vi "Remove and Rewire Objects_core.vi"(8 "error in (no error)":errorcluster, 11 "Items to Remove":refnum<vi>[](array[refnum])) -> (0 "error out":errorcluster, 3 "Any Items Removed?":bool)   [LabVIEW 2017]
uses:
  <vilib>/Utility/Data Type/Type Definitions/Data Type.ctl
  <vilib>/Utility/Data Type/NI_Data Type.lvlib
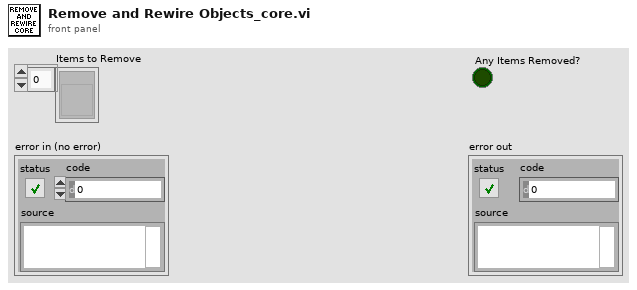
[diagram p1: front panel]
types:
  T1 = typedef "NI_Data Type.lvlib/Data Type.ctl" = enum8{"Invalid Type", "Void", "I8", "I16", "I32", "I64", "U8", "U16", "U32", "U64", "Single Float", "Double Float", "Extended Float", "Single Complex", "Double Complex", "Extended Complex", "Enum U8", "Enum U16", "Enum U32", "Enum U64", "Single Float With Unit", "Double Float With Unit", "Extended Float With Unit", "Single Complex with Unit", "Double Complex with Unit", "Extended Complex with Unit", "Boolean", "String", "Path", "Picture", "Tag", "Array", "Cluster", "Variant", "LV Variant", "Waveform", "Timestamp", "Digital Waveform", "Digital Data", "ExpressData", "Refnum", "External Data", "VI", "Poly VI", "LabVIEW Class Instance", "Fixed Point"}
  T2 = cluster{"Left":i32, "Top":i32, "Terminal":refnum<vi>}
  T3 = cluster{"Left":i32, "Top":i32, "Terminal":refnum<vi>}[]
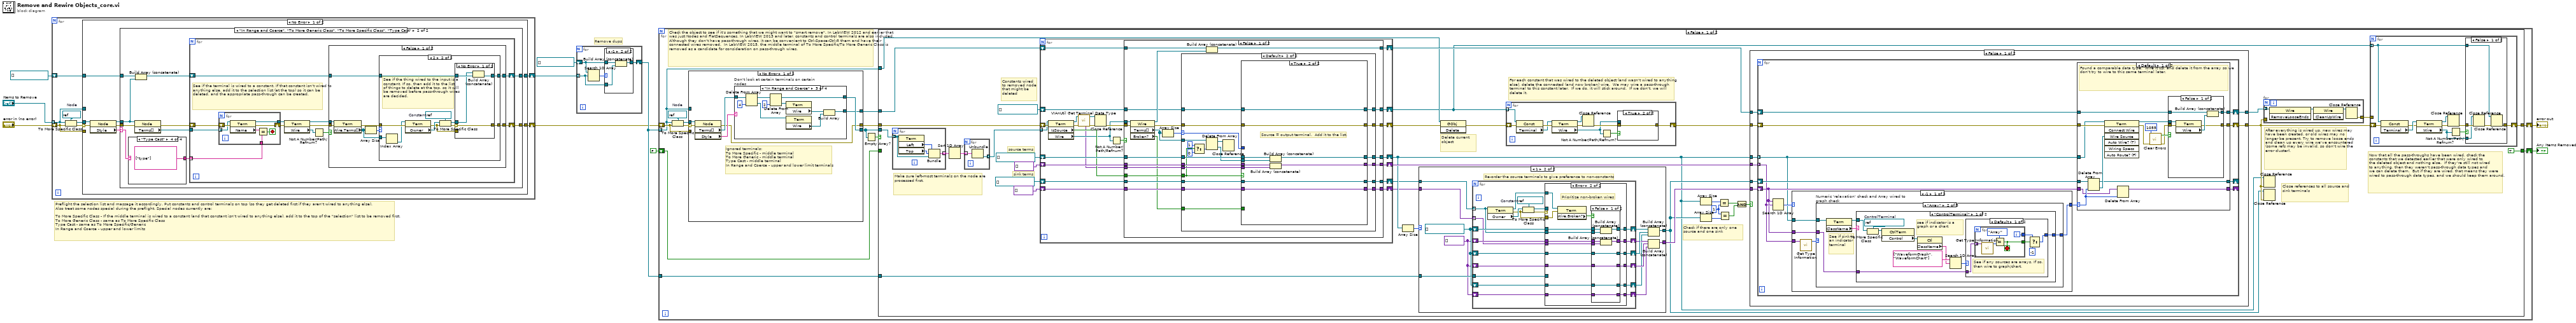
[diagram p0: block diagram]
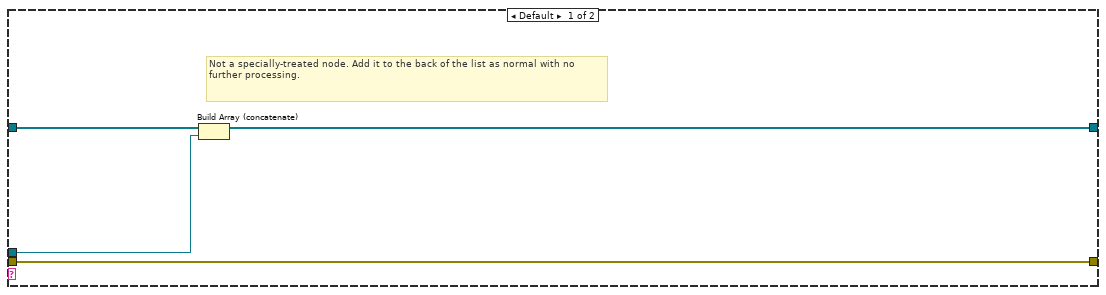
[diagram p3: hidden frame]
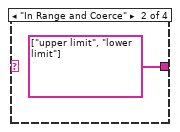
[diagram p5: hidden frame]
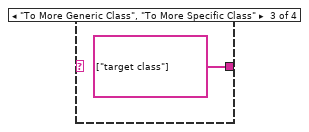
[diagram p6: hidden frame]
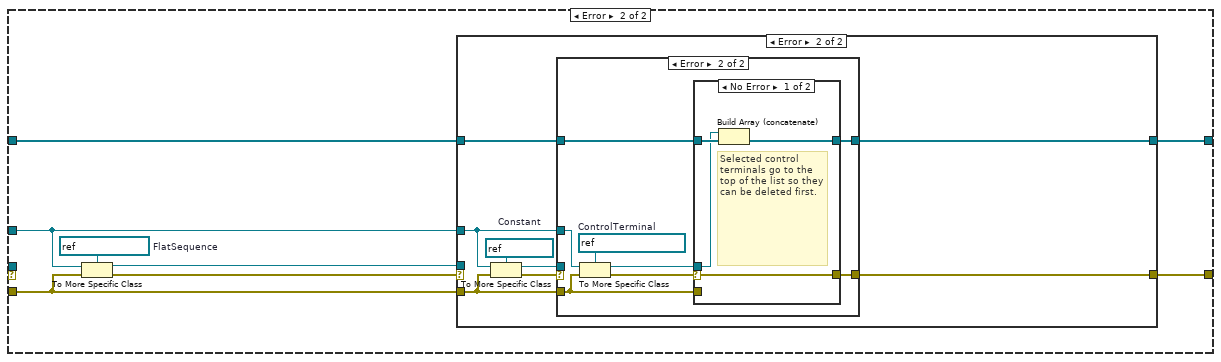
[diagram p10: hidden frame]
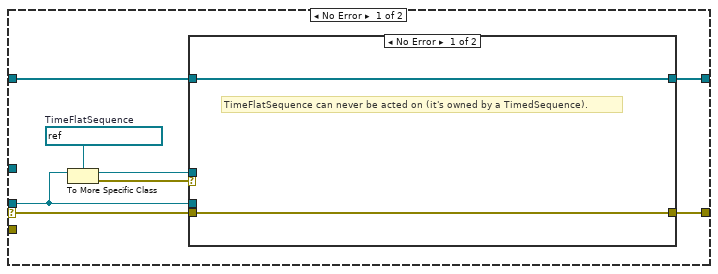
[diagram p11: hidden frame]
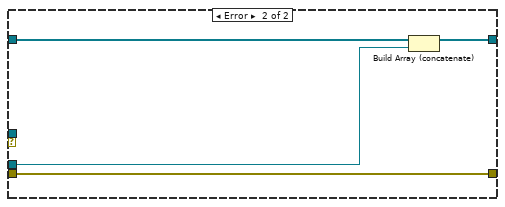
[diagram p12: hidden frame]
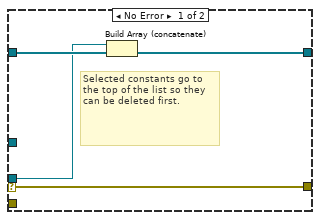
[diagram p13: hidden frame]
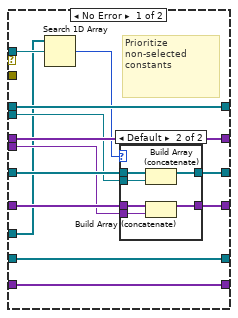
[diagram p16: hidden frame]
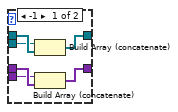
[diagram p17: hidden frame]
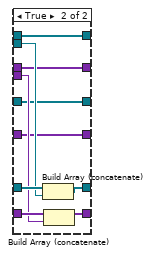
[diagram p18: hidden frame]
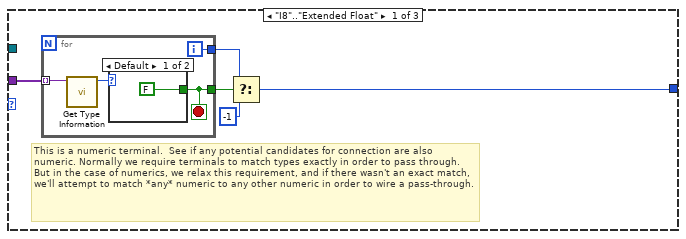
[diagram p19: hidden frame]
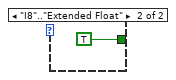
[diagram p20: hidden frame]
diagram:
  # "Preflight the selection list and massage it accordingly. Put constants and control terminals on top (so they get deleted first if they aren't wired to anything else).\nAlso treat some nodes special during the preflight. Special nodes currently are:\n\nTo More Specific Class - If the middle terminal is wired to a constant (and that constant isn't wired to anything else), add it to the top of the \"selection\" list to be removed first.\nTo More Generic Class - same as To More Specific Class\nType Cast - same as To More Specific/Generic\nIn Range and Coerce - upper and lower limits"
  # "Remove dups"
  n1 = for {
    tunnel: "Items to Remove" -> [w12] mode=indexing
    shift-right: [w13] -> w6
    shift-left: "error in (no error)" -> [w16]
    shift-right: [w14] -> w8
    shift-left: refnum<vi>[] [] ("SelList[]") -> [w15]
    w11 = refnum<vi> refnum  # Node
    n2 = To More Specific Class(target class=w11, reference=w12, error in=w16) -> (specific class reference=w18:refnum<vi>, error out=w17:errorcluster)
    n3 = case shown="No Error" w17 {
      selector: w17 -> [w26 _]
      tunnel: w18 -> [w25 _]
      tunnel: [w19 w97] -> w13
      tunnel: w12 -> [_ w95]
      tunnel: w16 -> [_ w96]
      tunnel: w15 -> [w21 w94]
      tunnel: [w20 w93] -> w14
      frame No Error {
        n4 = property class="Node"(reference=w25, error in=w26) -> (reference out=w22:refnum<vi>, error out=w23:errorcluster, "Style"=w24:string)
        n5 = case shown="\"In Range and Coerce\", \"To More Generic Class\", \"To More Specific Class\", \"Type Cast\"" w24 {
          selector: w24 -> [_ w31]
          tunnel: w23 -> [w28 w39]
          tunnel: w22 -> [w27 w38]
          tunnel: w21 -> [w30 w40]
          tunnel: [w29 w34] -> w20
          tunnel: [w28 w33] -> w19
          frame Default {
            # "Not a specially-treated node. Add it to the back of the list as normal with no further processing."
            n6 = Build Array (concatenate)(w30, w27) -> (w29:refnum<vi>[])
          }
          frame "In Range and Coerce", "To More Generic Class", "To More Specific Class", "Type Cast" {
            n7 = case shown="\"Type Cast\"" w31 {
              tunnel: [_ string[] ["upper limit", "lower limit"] string[] ["target class"] string[] ["type"]] -> w32
              frame Default {
              }
              frame "In Range and Coerce" {
              }
              frame "To More Generic Class", "To More Specific Class" {
              }
              frame "Type Cast" {
              }
            }
            n8 = property class="Node"(reference=w38, error in=w39) -> (error out=w37:errorcluster, "Terms[]"=w36:refnum<vi>[])  [unwired: 1 out]
            n9 = Build Array (concatenate)(w40, w38) -> (w35:refnum<vi>[])
            n10 = for {
              tunnel: w36 -> [w54]
              shift-right: [w50] -> w33
              shift-left: w37 -> [w55]
              shift-right: [w51] -> w34
              shift-left: w35 -> [w52]
              tunnel: w32 -> [w44] mode=indexing
              # "See if the terminal is wired to a constant. If that constant isn't wired to anything else, add it to the selection list (at the top) so it can be deleted, and the appropriate pass-through can be created."
              n11 = for {
                tunnel: w54 -> [w90] mode=indexing
                tunnel: [w88] -> w48
                shift-right: [w87] -> w53
                shift-left: w55 -> [w91]
                tunnel: w44 -> [w85]
                stop <- w86 stop-if-true
                n12 = property class="Term"(reference=w90, error in=w91) -> (reference out=w88:refnum<vi>, error out=w87:errorcluster, "Name"=w89:string)
                n13 = Equal?(x=w89, y=w85) -> (x = y?=w86:bool)
              }
              n14 = property class="Term"(reference=w48, error in=w53) -> (reference out=w47:refnum<vi>, error out=w49:errorcluster, "Wire"=w46:refnum<vi>)
              n15 = Not A Number/Path/Refnum?(number/path/refnum=w46) -> (NaN/Path/Refnum?=w45:bool)
              n16 = case shown="False" w45 {
                tunnel: w52 -> [w63 w84]
                tunnel: [w60 w84] -> w51
                tunnel: [w59 w83] -> w50
                tunnel: w49 -> [w57 w83]
                tunnel: w47 -> [w56 _]
                frame False {
                  n17 = property class="Term"(reference=w56, error in=w57) -> (error out=w62:errorcluster, "Wire.Terms[]"=w58:refnum<vi>[])  [unwired: 1 out]
                  n18 = Array Size(array=w58) -> (size(s)=w61:i32)
                  n19 = case shown="2" w61 {
                    tunnel: w63 -> [w65 w70]
                    tunnel: w62 -> [w64 w75]
                    tunnel: [w65 w69] -> w60
                    tunnel: [w64 w67] -> w59
                    tunnel: w58 -> [_ w76]
                    frame Default {
                      # "Any number of terminals on the upper/lower limit wires other than 2 means that whatever is wired to it, is also wired to something else. Don't try to delete that thing in this case."
                    }
                    frame 2 {
                      w72 = refnum<vi> refnum  # Constant
                      # "See if the thing wired to the input is a constant. If so, then add it to the list of things to delete at the top, so it will be removed before pass-through wires are decided."
                      n20 = Index Array(array=w76) -> (element=w74:refnum<vi>)  [unwired: 1 in]
                      n21 = property class="Term"(reference=w74, error in=w75) -> (error out=w68:errorcluster, "Owner"=w73:refnum<vi>)  [unwired: 1 out]
                      n22 = To More Specific Class(target class=w72, reference=w73, error in=w68) -> (specific class reference=w66:refnum<vi>, error out=w71:errorcluster)
                      n23 = case shown="No Error" w71 {
                        selector: w71 -> [w78 _]
                        tunnel: w70 -> [w80 w82]
                        tunnel: [w79 w82] -> w69
                        tunnel: w68 -> [_ w81]
                        tunnel: [w78 w81] -> w67
                        tunnel: w66 -> [w77 _]
                        frame No Error {
                          n24 = Build Array (concatenate)(w77, w80) -> (w79:refnum<vi>[])
                        }
                        frame Error {
                        }
                      }
                    }
                  }
                }
                frame True {
                  # "Terminal is not wired...no further work necessary"
                }
              }
            }
          }
        }
      }
      frame Error {
        w92 = refnum<vi> refnum  # FlatSequence
        n25 = To More Specific Class(target class=w92, reference=w95, error in=w96) -> (specific class reference=w98:refnum<vi>, error out=w99:errorcluster)
        n26 = case shown="Error" w99 {
          selector: w99 -> [w102 _]
          tunnel: w98 -> [w104 _]
          tunnel: [w101 w117] -> w97
          tunnel: w96 -> [_ w118]
          tunnel: w95 -> [_ w119]
          tunnel: w94 -> [w107 w116]
          tunnel: [w106 w115] -> w93
          frame No Error {
            w105 = refnum<vi> refnum  # TimeFlatSequence
            n27 = To More Specific Class(target class=w105, reference=w104) -> (specific class reference=w100:refnum<vi>, error out=w103:errorcluster)  [unwired: 1 in]
            n28 = case shown="No Error" w103 {
              tunnel: w107 -> [w108 w113]
              tunnel: [w108 w112] -> w106
              tunnel: w104 -> [_ w111]
              tunnel: w102 -> [w109 w110]
              tunnel: [w109 w110] -> w101
              tunnel: w100 -> [_ _]
              frame No Error {
                # "TimeFlatSequence can never be acted on (it's owned by a TimedSequence)."
              }
              frame Error {
                n29 = Build Array (concatenate)(w113, w111) -> (w112:refnum<vi>[])
              }
            }
          }
          frame Error {
            w114 = refnum<vi> refnum  # Constant
            n30 = To More Specific Class(target class=w114, reference=w119, error in=w118) -> (specific class reference=w120:refnum<vi>, error out=w121:errorcluster)
            n31 = case shown="Error" w121 {
              selector: w121 -> [w125 _]
              tunnel: w120 -> [w122 _]
              tunnel: w119 -> [_ w133]
              tunnel: w118 -> [_ w130]
              tunnel: [w125 w129] -> w117
              tunnel: w116 -> [w124 w128]
              tunnel: [w123 w127] -> w115
              frame No Error {
                # "Selected constants go to the top of the list so they can be deleted first."
                n32 = Build Array (concatenate)(w122, w124) -> (w123:refnum<vi>[])
              }
              frame Error {
                w126 = refnum<vi> refnum  # ControlTerminal
                n33 = To More Specific Class(target class=w126, reference=w133, error in=w130) -> (specific class reference=w131:refnum<vi>, error out=w132:errorcluster)
                n34 = case shown="No Error" w132 {
                  selector: w132 -> [w137 _]
                  tunnel: w131 -> [w134 _]
                  tunnel: w130 -> [_ w139]
                  tunnel: [w137 w139] -> w129
                  tunnel: w128 -> [w136 w138]
                  tunnel: [w135 w138] -> w127
                  frame No Error {
                    # "Selected control terminals go to the top of the list so they can be deleted first."
                    n35 = Build Array (concatenate)(w134, w136) -> (w135:refnum<vi>[])
                  }
                  frame Error {
                  }
                }
              }
            }
          }
        }
      }
    }
  }
  n36 = for {
    tunnel: w8 -> [w140] mode=indexing
    shift-right: [w141] -> w10
    shift-left: refnum<vi>[] [] ("SelList[]") -> [w142]
    n37 = Search 1D Array(1D array=w142, element=w140) -> (index of element=w143:i32)  [unwired: 1 in]
    n38 = case shown="-1" w143 {
      tunnel: w142 -> [w144 w147]
      tunnel: [w144 w146] -> w141
      tunnel: w140 -> [_ w145]
      frame Default {
      }
      frame -1 {
        n39 = Build Array (concatenate)(w147, w145) -> (w146:refnum<vi>[])
      }
    }
  }
  n40 = for {
    tunnel: w10 -> [w154] mode=indexing
    shift-right: [w153] -> w2
    shift-left: FALSE -> [w148]
    shift-right: [w152] -> w3
    shift-left: w6 -> [w158]
    tunnel: w10 -> [w151]
    w150 = refnum<vi> refnum  # Node
    # "Check the object to see if it's something that we might want to \"smart remove\". In LabVIEW 2012 and earlier that was just Nodes and FlatSequences. In LabVIEW 2013 and later, constants and control terminals are also included. Although they don't have pass-through wires, it can be convenient to Ctrl-Space-Ctrl-R them and have their connected wires removed.  In LabVIEW 2015, the middle terminal of To More Specific/To More Generic Class is removed as a candidate for consideration on pass-through wires."
    n41 = To More Specific Class(target class=w150, reference=w154, error in=w158) -> (specific class reference=w159:refnum<vi>, error out=w160:errorcluster)
    n42 = case shown="No Error" w160 {
      selector: w160 -> [w572 _]
      tunnel: w159 -> [w571 _]
      tunnel: [w568 w598] -> w155
      tunnel: [w566 w600] -> w156
      tunnel: w154 -> [_ w597]
      tunnel: w158 -> [_ w599]
      tunnel: [w567 _] -> w149
      frame No Error {
        # "Ignored terminals:\nTo More Specific - middle terminal\nTo More Generic - middle terminal\nType Cast - middle terminal\nIn Range and Coerce - upper and lower limit terminals"
        n43 = property class="Node"(reference=w571, error in=w572) -> (error out=w566:errorcluster, "Terms[]"=w569:refnum<vi>[], "Style"=w570:string)  [unwired: 1 out]
        n44 = case "Don't look at certain terminals on certain nodes" shown="\"In Range and Coerce\"" w570 {
          tunnel: w569 -> [w578 w584 w594 w595]
          tunnel: [w576 w582 w588 w595] -> w568
          tunnel: [w573 w579 w590 _] -> w567
          frame "To More Generic Class", "Type Cast" {
            n45 = Delete From Array(array=w578, index=1) -> (deleted portion=w574:refnum<vi>, array with subset deleted=w576:refnum<vi>[])  [unwired: 1 in]
            n46 = property class="Term"(reference=w574) -> ("Wire"=w575:refnum<vi>)  [unwired: 1 in, 2 out]
            n47 = Build Array(w575) -> (w573:refnum<vi>[])
          }
          frame "To More Specific Class" {
            n48 = Delete From Array(array=w584, index=2) -> (deleted portion=w580:refnum<vi>, array with subset deleted=w582:refnum<vi>[])  [unwired: 1 in]
            n49 = property class="Term"(reference=w580) -> ("Wire"=w581:refnum<vi>)  [unwired: 1 in, 2 out]
            n50 = Build Array(w581) -> (w579:refnum<vi>[])
          }
          frame "In Range and Coerce" {
            n51 = Delete From Array(array=w594, index=4) -> (deleted portion=w591:refnum<vi>, array with subset deleted=w589:refnum<vi>[])  [unwired: 1 in]
            n52 = Delete From Array(array=w589, index=2) -> (deleted portion=w586:refnum<vi>, array with subset deleted=w588:refnum<vi>[])  [unwired: 1 in]
            n53 = property class="Term"(reference=w586) -> ("Wire"=w585:refnum<vi>)  [unwired: 1 in, 2 out]
            n54 = property class="Term"(reference=w591) -> ("Wire"=w592:refnum<vi>)  [unwired: 1 in, 2 out]
            n55 = Build Array(w585, w592) -> (w590:refnum<vi>[])
          }
          frame Default {
          }
        }
      }
      frame Error {
        w596 = refnum<vi> refnum  # FlatSequence
        n56 = To More Specific Class(target class=w596, reference=w597, error in=w599) -> (specific class reference=w601:refnum<vi>, error out=w602:errorcluster)
        n57 = case shown="Error" w602 {
          selector: w602 -> [w606 _]
          tunnel: w601 -> [w605 _]
          tunnel: [w604 w608] -> w600
          tunnel: w599 -> [_ w610]
          tunnel: [w603 w609] -> w598
          tunnel: w597 -> [_ w611]
          frame No Error {
            n58 = property class="FlatSeq"(reference=w605, error in=w606) -> (error out=w604:errorcluster, "Terms[]"=w603:refnum<vi>[])  [unwired: 1 out]
          }
          frame Error {
            w607 = refnum<vi> refnum  # Constant
            n59 = To More Specific Class(target class=w607, reference=w611, error in=w610) -> (specific class reference=w612:refnum<vi>, error out=w613:errorcluster)
            n60 = case shown="Error" w613 {
              selector: w613 -> [w617 _]
              tunnel: w612 -> [w618 _]
              tunnel: w611 -> [_ w625]
              tunnel: w610 -> [_ w622]
              tunnel: [w615 w620] -> w609
              tunnel: [w614 w621] -> w608
              frame No Error {
                n61 = property class="Const"(reference=w618, error in=w617) -> (error out=w614:errorcluster, "Terminal"=w616:refnum<vi>)  [unwired: 1 out]
                n62 = Build Array(w616) -> (w615:refnum<vi>[])
              }
              frame Error {
                w619 = refnum<vi> refnum  # ControlTerminal
                n63 = To More Specific Class(target class=w619, reference=w625, error in=w622) -> (specific class reference=w623:refnum<vi>, error out=w624:errorcluster)
                n64 = case shown="No Error" w624 {
                  selector: w624 -> [w628 _]
                  tunnel: w623 -> [w627 _]
                  tunnel: w622 -> [_ w629]
                  tunnel: [w628 w629] -> w621
                  tunnel: [w626 _] -> w620
                  frame No Error {
                    n65 = Build Array(w627) -> (w626:refnum<vi>[])
                  }
                  frame Error {
                  }
                }
              }
            }
          }
        }
      }
    }
    n66 = Empty Array?(array=w155) -> (empty?=w157:bool)
    n67 = case shown="False" w157 {
      tunnel: w156 -> [w196 w565]
      tunnel: [w182 w565] -> w152
      tunnel: w148 -> [_ w564]
      tunnel: w155 -> [w163 _]
      tunnel: w154 -> [w186 _]
      tunnel: [TRUE w564] -> w153
      tunnel: w151 -> [w168 _]
      tunnel: w149 -> [w161 _]
      frame False {
        w177 = 1 ("y")
        # "Make sure left-most terminals on the node are processed first."
        # "Check if there are only one source and one sink"
        # "Now that all the pass-throughs have been wired, check the\nconstants that we detected earlier that were only wired to\nthe deleted object and nothing else.  If they're still not wired\nto anything, then they weren't pass-through data types and\nwe can delete them.  But if they are wired, that means they were\nwired to pass-through data types, and we should keep them around."
        # "For each constant that was wired to the deleted object (and wasn't wired to anything\nelse), delete the connected (and now broken) wire.  We may wire a pass-through\nterminal to this constant later.  If we do, it will stick around.  If we don't, we will\ndelete it."
        # "Constants wired\nto removed node\nthat might be\ndeleted"
        # "After everything is wired up, new wires may have been created, or old wires may no longer be present. Try to remove loose ends and clean up every wire we've encountered (some refs may be invalid, so don't wire the error cluster)."
        # "Close references to all source and\nsink terminals"
        # "Delete current object"
        # "sink terms"
        # "source terms"
        n68 = for {
          tunnel: w163 -> [w200] mode=indexing
          tunnel: [w201] -> w165 mode=indexing
          n69 = property class="Term"(reference=w200) -> ("Left"=w202:i32, "Top"=w199:i32)  [unwired: 1 in, 2 out]
          n70 = Bundle("Left"=w202, "Top"=w199, "Terminal"=w200) -> (w201:T2)  [unwired: 1 in]
        }
        n71 = Sort 1D Array(array=w165) -> (sorted array=w164:T3)
        n72 = for {
          tunnel: w164 -> [w198] mode=indexing
          tunnel: [w197] -> w162 mode=indexing
          n73 = Unbundle(w198) -> ("Terminal"=w197:refnum<vi>)  [unwired: 2 out]
        }
        n74 = for {
          shift-right: [w451] -> w190
          shift-left: w196 -> [w463]
          tunnel: w162 -> [w462] mode=indexing
          shift-right: [w455] -> w170
          shift-left: refnum<vi>[] [] -> [w461]
          shift-right: [w454] -> w173
          shift-left: variant[] [] -> [w460]
          shift-right: [w457] -> w167
          shift-left: refnum<vi>[] [] -> [w459]
          shift-right: [w456] -> w166
          shift-left: variant[] [] -> [w458]
          shift-right: [w447] -> w189
          shift-left: w161 -> [w448]
          shift-right: [w445] -> w180
          shift-left: refnum<vi>[] [] -> [w446]
          n75 = property class="Term"(reference=w462, error in=w463) -> (reference out=w442:refnum<vi>, error out=w444:errorcluster, "IsSource"=w452:bool, "Wire"=w450:refnum<vi>)
          n76 = call <vilib>:"VIAnUtil Get Terminal Data Type.vi"("error in (no error)"=w444, "Terminal"=w442) -> ("error out"=w443:errorcluster, "dup  Terminal"=w441:refnum<vi>, "Type Variant"=w440:variant)  [unwired: 6 in, 1 out]
          n77 = Close Reference(reference=w441, error in (no error)=w443) -> (error out=w453:errorcluster)
          n78 = Not A Number/Path/Refnum?(number/path/refnum=w450) -> (NaN/Path/Refnum?=w449:bool)
          n79 = case shown="False" w449 {
            tunnel: w461 -> [w485 w561]
            tunnel: w460 -> [w484 w560]
            tunnel: w459 -> [w483 w559]
            tunnel: w458 -> [w482 w558]
            tunnel: w440 -> [w481 _]
            tunnel: [w480 w559] -> w457
            tunnel: [w479 w558] -> w456
            tunnel: [w478 w561] -> w455
            tunnel: [w477 w560] -> w454
            tunnel: w453 -> [w476 w562]
            tunnel: w452 -> [w474 _]
            tunnel: [w468 w562] -> w451
            tunnel: w450 -> [w475 _]
            tunnel: w448 -> [w473 w563]
            tunnel: [w472 w563] -> w447
            tunnel: w446 -> [w469 w557]
            tunnel: [w467 w557] -> w445
            frame False {
              n80 = property class="Wire"(reference=w475, error in=w476) -> (reference out=w471:refnum<vi>, error out=w470:errorcluster, "Terms[]"=w466:refnum<vi>[], "Broken?"=w464:bool)
              n81 = Array Size(array=w466) -> (size(s)=w465:i32)
              n82 = case shown="Default" w465 {
                selector: w465 -> [_ w494]
                tunnel: w485 -> [w489 w514]
                tunnel: w484 -> [w490 w513]
                tunnel: w483 -> [w491 w512]
                tunnel: w482 -> [w492 w511]
                tunnel: w481 -> [_ w510]
                tunnel: [w491 w509] -> w480
                tunnel: [w492 w508] -> w479
                tunnel: [w489 w507] -> w478
                tunnel: [w490 w506] -> w477
                tunnel: w474 -> [_ w500]
                tunnel: w470 -> [w486 w499]
                tunnel: w469 -> [w488 w498]
                tunnel: [w486 w497] -> w468
                tunnel: [w488 w496] -> w467
                tunnel: w466 -> [w487 w495]
                tunnel: w464 -> [_ w493]
                frame 1 {
                  # "If the wire only has one terminal, then it is a broken wire, with either no source\nor no sink.  Don't try to get data type information on this wire, as it will end up\nbeing removed by the \"Remove Loose Ends\" call later (note that we're still adding\nthe wire to the wires array above)."
                  n83 = Close Reference(reference=w487) -> ()  [unwired: 1 in, 1 out]
                }
                frame Default {
                  n84 = Select(t=1, s=w500, f=0) -> (s? t:f=w503:i32)
                  n85 = Delete From Array(array=w495, index=w503) -> (deleted portion=w501:refnum<vi>, array with subset deleted=w502:refnum<vi>[])  [unwired: 1 in]
                  n86 = Close Reference(reference=w502) -> ()  [unwired: 1 in, 1 out]
                  n87 = case shown="True" w500 {
                    tunnel: w514 -> [w533 w554]
                    tunnel: w513 -> [w532 w552]
                    tunnel: w512 -> [w535 w556]
                    tunnel: w511 -> [w534 w555]
                    tunnel: w510 -> [w518 w549]
                    tunnel: w501 -> [w521 w553]
                    tunnel: [w531 w556] -> w509
                    tunnel: [w530 w555] -> w508
                    tunnel: [w533 w551] -> w507
                    tunnel: [w532 w550] -> w506
                    tunnel: w499 -> [w529 w548]
                    tunnel: w498 -> [w523 w547]
                    tunnel: [w524 w548] -> w497
                    tunnel: [w522 w547] -> w496
                    tunnel: w494 -> [w520 _]
                    tunnel: w493 -> [w519 _]
                    frame False {
                      w515 = refnum<vi> refnum  # Constant
                      # "If wire was broken, use data type of source term (instead of sink on removed item) when trying to make a match later."
                      # "Sink = input terminal.  Add it to the list, and if it's wired to a constant, add that to the list of constants to potentially delete.  Except if the constant is wired to something else... in that case, keep the const."
                      n88 = property class="Term"(reference=w521, error in=w529) -> (error out=w525:errorcluster, "Owner"=w528:refnum<vi>, "Data Type"=w516:variant)  [unwired: 1 out]
                      n89 = Select(t=w516, s=w519, f=w518) -> (s? t:f=w517:variant)
                      n90 = To More Specific Class(target class=w515, reference=w528, error in=w525) -> (specific class reference=w526:refnum<vi>, error out=w527:errorcluster)
                      n91 = case shown="No Error" w527 {
                        selector: w527 -> [w538 _]
                        tunnel: w526 -> [w537 _]
                        tunnel: w525 -> [_ w546]
                        tunnel: [w538 w546] -> w524
                        tunnel: [w539 w545] -> w522
                        tunnel: w523 -> [w540 w545]
                        tunnel: w520 -> [w536 _]
                        frame No Error {
                          n92 = case shown="..2" w536 {
                            tunnel: w540 -> [w541 w544]
                            tunnel: [w541 w543] -> w539
                            tunnel: w537 -> [_ w542]
                            frame 3.. {
                            }
                            frame ..2 {
                              n93 = Build Array (concatenate)(w544, w542) -> (w543:refnum<vi>[])
                            }
                          }
                        }
                        frame Error {
                        }
                      }
                      n94 = Build Array (concatenate)(w535, w521) -> (w531:refnum<vi>[])
                      n95 = Build Array (concatenate)(w534, w517) -> (w530:variant[])
                    }
                    frame True {
                      # "Source = output terminal.  Add it to the list."
                      n96 = Build Array (concatenate)(w554, w553) -> (w551:refnum<vi>[])
                      n97 = Build Array (concatenate)(w552, w549) -> (w550:variant[])
                    }
                  }
                }
              }
              n98 = Build Array (concatenate)(w473, w471) -> (w472:refnum<vi>[])
            }
            frame True {
              # "This terminal isn't wired to anything.  Ignore it."
            }
          }
        }
        n99 = Array Size(array=w170) -> (size(s)=w169:i32)
        n100 = case shown="1" w169 {
          tunnel: w167 -> [w204 w217]
          tunnel: w166 -> [w203 w216]
          tunnel: [w203 w215] -> w172
          tunnel: [w204 w214] -> w171
          tunnel: w168 -> [_ w209]
          frame Default {
          }
          frame 1 {
            w207 = variant[] []
            w208 = refnum<vi>[] []
            # "Re-order the source terminals to give preference to non-constants"
            n101 = for {
              tunnel: w217 -> [w229] mode=indexing
              tunnel: w216 -> [w230] mode=indexing
              shift-right: [w232] -> w213
              shift-left: w208 -> [w234]
              shift-right: [w231] -> w211
              shift-left: w207 -> [w233]
              shift-right: [w227] -> w212
              shift-left: w208 -> [w228]
              shift-right: [w225] -> w210
              shift-left: w207 -> [w226]
              tunnel: w209 -> [w224]
              shift-right: [w219] -> w206
              shift-left: w208 -> [w221]
              shift-right: [w218] -> w205
              shift-left: w207 -> [w220]
              w237 = refnum<vi> refnum  # Constant
              n102 = property class="Term"(reference=w229) -> (reference out=w223:refnum<vi>, error out=w222:errorcluster, "Owner"=w238:refnum<vi>)  [unwired: 1 in]
              n103 = To More Specific Class(target class=w237, reference=w238, error in=w222) -> (specific class reference=w235:refnum<vi>, error out=w236:errorcluster)
              n104 = case shown="Error" w236 {
                tunnel: w235 -> [w243 _]
                tunnel: w234 -> [w251 w280]
                tunnel: w233 -> [w250 w279]
                tunnel: [w251 w278] -> w232
                tunnel: [w250 w277] -> w231
                tunnel: w230 -> [w244 w276]
                tunnel: w229 -> [w248 w275]
                tunnel: [w247 w266] -> w227
                tunnel: w228 -> [w249 w267]
                tunnel: w226 -> [w246 w265]
                tunnel: [w245 w264] -> w225
                tunnel: w224 -> [w242 _]
                tunnel: w223 -> [_ w273]
                tunnel: w222 -> [_ w274]
                tunnel: w221 -> [w240 w270]
                tunnel: w220 -> [w239 w268]
                tunnel: [w240 w271] -> w219
                tunnel: [w239 w269] -> w218
                frame No Error {
                  # "Prioritize non-selected constants"
                  n105 = Search 1D Array(1D array=w242, element=w243) -> (index of element=w241:i32)  [unwired: 1 in]
                  n106 = case shown="Default" w241 {
                    tunnel: w249 -> [w257 w263]
                    tunnel: w248 -> [w256 w262]
                    tunnel: [w255 w261] -> w247
                    tunnel: w246 -> [w254 w260]
                    tunnel: [w253 w259] -> w245
                    tunnel: w244 -> [w252 w258]
                    frame -1 {
                      n107 = Build Array (concatenate)(w256, w257) -> (w255:refnum<vi>[])
                      n108 = Build Array (concatenate)(w252, w254) -> (w253:variant[])
                    }
                    frame Default {
                      n109 = Build Array (concatenate)(w263, w262) -> (w261:refnum<vi>[])
                      n110 = Build Array (concatenate)(w260, w258) -> (w259:variant[])
                    }
                  }
                }
                frame Error {
                  # "Prioritize non-broken wires"
                  n111 = property class="Term"(reference=w273, error in=w274) -> ("Wire.Broken?"=w272:bool)  [unwired: 2 out]
                  n112 = case shown="False" w272 {
                    tunnel: w280 -> [w290 w294]
                    tunnel: w279 -> [w287 w293]
                    tunnel: [w289 w294] -> w278
                    tunnel: [w286 w293] -> w277
                    tunnel: w276 -> [w285 w295]
                    tunnel: w275 -> [w288 w298]
                    tunnel: [w284 w300] -> w271
                    tunnel: w270 -> [w284 w299]
                    tunnel: [w283 w297] -> w269
                    tunnel: w268 -> [w283 w296]
                    tunnel: w267 -> [w282 w292]
                    tunnel: [w282 w292] -> w266
                    tunnel: w265 -> [w281 w291]
                    tunnel: [w281 w291] -> w264
                    frame False {
                      n113 = Build Array (concatenate)(w290, w288) -> (w289:refnum<vi>[])
                      n114 = Build Array (concatenate)(w287, w285) -> (w286:variant[])
                    }
                    frame True {
                      n115 = Build Array (concatenate)(w299, w298) -> (w300:refnum<vi>[])
                      n116 = Build Array (concatenate)(w296, w295) -> (w297:variant[])
                    }
                  }
                }
              }
            }
            n117 = Build Array (concatenate)(w213, w212, w206) -> (w214:refnum<vi>[])
            n118 = Build Array (concatenate)(w211, w210, w205) -> (w215:variant[])
          }
        }
        n119 = invoke class="GObj" method="Delete"(reference=w186, error in=w190) -> (error out=w185:errorcluster)  [unwired: 1 in, 2 out]
        n120 = for {
          tunnel: w180 -> [w430] mode=indexing
          shift-right: [w424] -> w184
          shift-left: w185 -> [w431]
          n121 = property class="Const"(reference=w430, error in=w431) -> (error out=w429:errorcluster, "Terminal"=w428:refnum<vi>)  [unwired: 1 out]
          n122 = property class="Term"(reference=w428, error in=w429) -> (reference out=w426:refnum<vi>, error out=w427:errorcluster, "Wire"=w423:refnum<vi>)
          n123 = Close Reference(reference=w426, error in (no error)=w427) -> (error out=w425:errorcluster)
          n124 = Not A Number/Path/Refnum?(number/path/refnum=w423) -> (NaN/Path/Refnum?=w422:bool)
          n125 = case shown="True" w422 {
            tunnel: w425 -> [w434 w435]
            tunnel: [w433 w435] -> w424
            tunnel: w423 -> [w432 _]
            frame False {
              n126 = invoke class="Wire" method="Delete"(reference=w432, error in=w434) -> (error out=w433:errorcluster)  [unwired: 1 in, 2 out]
            }
            frame True {
            }
          }
        }
        n127 = Array Size(array=w170) -> (size(s)=w179:i32)
        n128 = Array Size(array=w171) -> (size(s)=w178:i32)
        n129 = Equal?(x=w179, y=w177) -> (x = y?=w176:bool)
        n130 = Equal?(x=w177, y=w178) -> (x = y?=w175:bool)
        n131 = And(x=w176, y=w175) -> (x .and. y?=w174:bool)
        n132 = case shown="False" w174 {
          tunnel: w173 -> [w308 _]
          tunnel: w172 -> [w307 _]
          tunnel: w189 -> [w306 w395]
          tunnel: [w305 w393] -> w188
          tunnel: w184 -> [w304 w401]
          tunnel: [w303 w396] -> w183
          tunnel: w170 -> [w302 w403]
          tunnel: w171 -> [w301 w402]
          frame False {
            n133 = for {
              shift-right: [w316] -> w303
              shift-left: w304 -> [w318]
              tunnel: w302 -> [w309] mode=indexing
              tunnel: w308 -> [w311] mode=indexing
              shift-right: [w319] -> w305
              shift-left: w306 -> [w320]
              shift-right: [w315] -> _
              shift-left: w301 -> [w317]
              shift-right: [w314] -> _
              shift-left: w307 -> [w310]
              n134 = Search 1D Array(1D array=w310, element=w311) -> (index of element=w313:i32)  [unwired: 1 in]
              n135 = case shown="-1" w313 {
                selector: w313 -> [_ w364]
                tunnel: [w322 w364] -> w312
                tunnel: w311 -> [w325 _]
                tunnel: w310 -> [w323 _]
                tunnel: w309 -> [w321 _]
                frame -1 {
                  n136 = call <vilib>:"Get Type Information.vi"("Variant"=w325) -> ("Type"=w324:T1)  [unwired: 6 in, 4 out]
                  n137 = case "Numeric 'relaxation' check and Array wired to graph check" shown="\"Array\"" w324 {
                    tunnel: w323 -> [w330 w337 _]
                    tunnel: [w326 w340 -1] -> w322
                    tunnel: w321 -> [_ w341 _]
                    frame "I8".."Extended Float" {
                      # "This is a numeric terminal.  See if any potential candidates for connection are also numeric. Normally we require terminals to match types exactly in order to pass through.  But in the case of numerics, we relax this requirement, and if there wasn't an exact match, we'll attempt to match *any* numeric to any other numeric in order to wire a pass-through."
                      n138 = for {
                        tunnel: w330 -> [w334] mode=indexing
                        tunnel: [w332] -> w329
                        tunnel: [w331] -> w328
                        i -> [w331]
                        stop <- w332 stop-if-true
                        n139 = call <vilib>:"Get Type Information.vi"("Variant"=w334) -> ("Type"=w333:T1)  [unwired: 6 in, 4 out]
                        n140 = case shown="Default" w333 {
                          tunnel: [FALSE TRUE] -> w332
                          frame Default {
                          }
                          frame "I8".."Extended Float" {
                          }
                        }
                      }
                      n141 = Select(t=w328, s=w329, f=-1) -> (s? t:f=w326:i32)
                    }
                    frame "Array" {
                      # "See if sink is an indicator terminal"
                      n142 = property class="Term"(reference=w341) -> (reference out=w338:refnum<vi>, "ClassName"=w339:string)  [unwired: 1 in, 1 out]
                      n143 = case shown="\"ControlTerminal\"" w339 {
                        tunnel: [w343 -1] -> w340
                        tunnel: w338 -> [w350 _]
                        tunnel: w337 -> [w342 _]
                        frame "ControlTerminal" {
                          w349 = refnum<vi> refnum  # ControlTerminal
                          # "see if indicator is a graph or a chart"
                          n144 = To More Specific Class(target class=w349, reference=w350) -> (specific class reference=w348:refnum<vi>)  [unwired: 1 in, 1 out]
                          n145 = property class="CtrlTerm"(reference=w348) -> ("Control"=w347:refnum<vi>)  [unwired: 1 in, 2 out]
                          n146 = property class="Ctl"(reference=w347) -> ("ClassName"=w345:string)  [unwired: 1 in, 2 out]
                          n147 = Search 1D Array(1D array=string[] ["WaveformGraph", "WaveformChart"], element=w345) -> (index of element=w344:i32)  [unwired: 1 in]
                          n148 = case shown="Default" w344 {
                            tunnel: [w352 -1] -> w343
                            tunnel: w342 -> [w355 _]
                            frame Default {
                              # "See if any sources are arrays. If so, then wire to graph/chart."
                              n149 = for {
                                tunnel: w355 -> [w360] mode=indexing
                                tunnel: [w357] -> w354
                                tunnel: [w356] -> w353
                                i -> [w356]
                                stop <- w357 stop-if-true
                                n150 = call <vilib>:"Get Type Information.vi"("Variant"=w360) -> ("Type"=w359:T1)  [unwired: 6 in, 4 out]
                                n151 = Equal?(x=Data_Type."Array", y=w359) -> (x = y?=w357:bool)
                              }
                              n152 = Select(t=w353, s=w354, f=-1) -> (s? t:f=w352:i32)
                            }
                            frame -1 {
                              # "Wired terminal is not a graph or chart"
                            }
                          }
                        }
                        frame Default {
                          # "The terminal is not an indicator terminal. This is not a graph/chart sink."
                        }
                      }
                    }
                    frame Default {
                      # "Not a numeric type or an array that might be wired to a chart/graph.\nDon't try to 'relax' it."
                    }
                  }
                }
                frame Default {
                  # "Exact match was found.  Use it."
                }
              }
              n153 = case shown="Default" w312 {
                selector: w312 -> [w370 _]
                tunnel: w320 -> [w375 w392]
                tunnel: [w374 w392] -> w319
                tunnel: w318 -> [w379 w391]
                tunnel: w309 -> [w378 _]
                tunnel: w317 -> [w380 w390]
                tunnel: [w373 w391] -> w316
                tunnel: [w372 w390] -> w315
                tunnel: w310 -> [w369 w389]
                tunnel: [w371 w389] -> w314
                frame Default {
                  # "Found a comparable data type.  Wire it up, and delete it from the array so we don't try to wire to this same terminal later."
                  n154 = Delete From Array(array=w380, index=w370) -> (deleted portion=w377:refnum<vi>, array with subset deleted=w372:refnum<vi>[])  [unwired: 1 in]
                  n155 = invoke class="Term" method="Connect Wire"(reference=w378, error in=w379, "Wire Source"=w377) -> (reference out=w376:refnum<vi>, error out=w366:errorcluster)  [unwired: 4 in, 5 out]
                  n156 = Delete From Array(array=w369, index=w370) -> (array with subset deleted=w371:variant[])  [unwired: 1 in, 1 out]
                  n157 = call <vilib>:"Clear Errors.vi"("error in (no error)"=w366, "specific error code to clear (0: all)"=1055) -> ("error out"=w365:errorcluster, "specific error cleared?"=w367:bool)  [unwired: 4 in]
                  n158 = case shown="False" w367 {
                    tunnel: w376 -> [w386 _]
                    tunnel: w375 -> [w385 w388]
                    tunnel: [w383 w388] -> w374
                    tunnel: [w382 w387] -> w373
                    tunnel: w365 -> [w381 w387]
                    frame False {
                      n159 = property class="Term"(reference=w386, error in=w381) -> (error out=w382:errorcluster, "Wire"=w384:refnum<vi>)  [unwired: 1 out]
                      n160 = Build Array (concatenate)(w385, w384) -> (w383:refnum<vi>[])
                    }
                    frame True {
                      # "One of the terminal references became invalid. This is usually when the removed node was wired to a source that disappeared (like an unsourced tunnel)."
                    }
                  }
                }
                frame -1 {
                  # "No comparable data type found for this item. Don't try to wire it up."
                }
              }
            }
          }
          frame True {
            # "If there is only one source and one sink, go ahead and wire them up, don't bother doing the data type check. This solves the problem where there was originally a broken wire because data types didn't match, and the mismatch caused us to not try to rewire the source and sink."
            n161 = Index Array(array=w403) -> (element=w400:refnum<vi>)  [unwired: 1 in]
            n162 = Index Array(array=w402) -> (element=w399:refnum<vi>)  [unwired: 1 in]
            n163 = invoke class="Term" method="Connect Wire"(reference=w400, error in=w401, "Wire Source"=w399) -> (reference out=w398:refnum<vi>, error out=w397:errorcluster)  [unwired: 4 in, 5 out]
            n164 = property class="Term"(reference=w398, error in=w397) -> (error out=w396:errorcluster, "Wire"=w394:refnum<vi>)  [unwired: 1 out]
            n165 = Build Array (concatenate)(w395, w394) -> (w393:refnum<vi>[])
          }
        }
        n166 = for {
          tunnel: w188 -> [w439] mode=indexing
          tunnel: w183 -> [_]
          tunnel: [w436] -> w181
          n167 = invoke class="Wire" method="RemoveLooseEnds"(reference=w439) -> (reference out=w438:refnum<vi>)  [unwired: 2 in, 2 out]
          n168 = invoke class="Wire" method="CleanUpWire"(reference=w438) -> (reference out=w437:refnum<vi>)  [unwired: 2 in, 2 out]
          n169 = Close Reference(reference=w437) -> (error out=w436:errorcluster)  [unwired: 1 in]
        }
        n170 = Close Reference(reference=w170, error in (no error)=w183) -> ()  [unwired: 1 out]
        n171 = Close Reference(reference=w171, error in (no error)=w183) -> ()  [unwired: 1 out]
        n172 = for {
          shift-right: [w404] -> w182
          shift-left: w183 -> [w409]
          tunnel: w181 -> [_]
          tunnel: w180 -> [w406] mode=indexing
          n173 = property class="Const"(reference=w406, error in=w409) -> (error out=w410:errorcluster, "Terminal"=w411:refnum<vi>)  [unwired: 1 out]
          n174 = property class="Term"(reference=w411, error in=w410) -> (reference out=w413:refnum<vi>, error out=w412:errorcluster, "Wire"=w405:refnum<vi>)
          n175 = Close Reference(reference=w413, error in (no error)=w412) -> (error out=w407:errorcluster)
          n176 = Not A Number/Path/Refnum?(number/path/refnum=w405) -> (NaN/Path/Refnum?=w408:bool)
          n177 = case shown="False" w408 {
            tunnel: w407 -> [w418 w420]
            tunnel: w406 -> [w414 w419]
            tunnel: w405 -> [w417 _]
            tunnel: [w415 w421] -> w404
            frame False {
              n178 = Close Reference(reference=w417, error in (no error)=w418) -> (error out=w416:errorcluster)
              n179 = Close Reference(reference=w414, error in (no error)=w416) -> (error out=w415:errorcluster)
            }
            frame True {
              n180 = invoke class="Const" method="Delete"(reference=w419, error in=w420) -> (error out=w421:errorcluster)  [unwired: 1 in, 2 out]
            }
          }
        }
      }
      frame True {
        # "Invalid object class, ignore this item."
      }
    }
  }
  "error out" <- w3
  "Any Items Removed?" <- w2
